vi "Chunked Streaming.vi"(8 "error in (no error)":errorcluster, 9 "Stream in":refnum<k5>, 11 "Streamable Response in":refnum<class "Streamable Response.lvclass">) -> (0 "error out":errorcluster, 1 "Stream out":refnum<k5>, 3 "Streamable Response out":refnum<class "Streamable Response.lvclass">)   [LabVIEW 2020, in "HTTP Utils.lvlib" / "Streamable Response.lvclass"]
uses:
  Streamable Response.lvclass
  Streamable Response.lvclass/Streamable Response.ctl
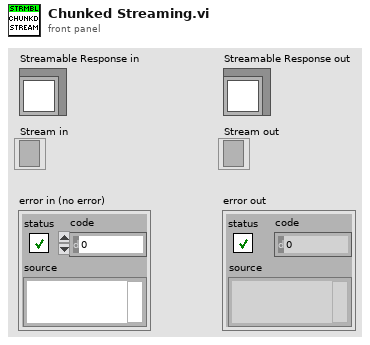
[diagram p1: front panel]
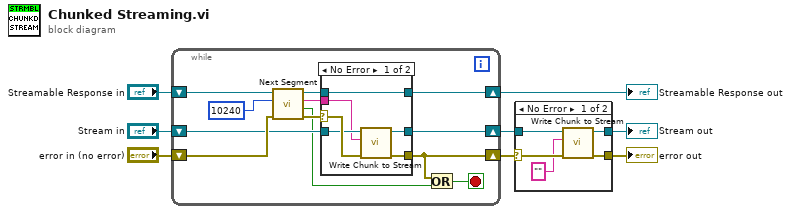
[diagram p0: block diagram]
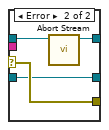
[diagram p3: hidden frame]
diagram:
  n1 = while {
    shift-right: [w15] -> w7
    shift-left: "Streamable Response in" -> [w20]
    shift-right: [w11] -> w4
    shift-left: "error in (no error)" -> [w18]
    shift-right: [w12] -> w3
    shift-left: "Stream in" -> [w14]
    stop <- w9 stop-if-true
    n2 = call-dynamic "Next Segment.vi"("error in (no error)"=w18, "Count"=10240, "Streamable Response in"=w20) -> ("error out"=w17:errorcluster, "Last?"=w10:bool, "Data"=w13:string, "Streamable Response out"=w16:refnum<class "Streamable Response.lvclass">)  [unwired: 5 in]
    n3 = case shown="No Error" w17 {
      selector: w17 -> [w26 w28]
      tunnel: w16 -> [w25 w30]
      tunnel: [w25 w29] -> w15
      tunnel: [w21 w28] -> w11
      tunnel: w14 -> [w24 w27]
      tunnel: w13 -> [w22 _]
      tunnel: [w23 w27] -> w12
      frame No Error {
        n4 = call "Write Chunk to Stream.vi"("error in (no error)"=w26, "Chunk"=w22, "Stream in"=w24) -> ("error out"=w21:errorcluster, "Stream out"=w23:refnum<k5>)  [unwired: 7 in]
      }
      frame Error {
        n5 = call-dynamic "Abort Stream.vi"("Streamable Response in"=w30) -> ("Streamable Response out"=w29:refnum<class "Streamable Response.lvclass">)  [unwired: 9 in, 1 out]
      }
    }
    n6 = Or(x=w11, y=w10) -> (x .or. y?=w9:bool)
  }
  "Streamable Response out" <- w7
  n7 = case shown="No Error" w4 {
    selector: w4 -> [w34 w36]
    tunnel: w3 -> [w35 w37]
    tunnel: [w32 w37] -> w2
    tunnel: [w31 w36] -> w1
    frame No Error {
      n8 = call "Write Chunk to Stream.vi"("error in (no error)"=w34, "Chunk"="", "Stream in"=w35) -> ("error out"=w31:errorcluster, "Stream out"=w32:refnum<k5>)  [unwired: 7 in]
    }
    frame Error {
    }
  }
  "error out" <- w1
  "Stream out" <- w2
